vi "Periodic Tasks.vi"(0 "error in":errorcluster) -> ()   [LabVIEW 2019]
doc: "All TeleOperated, Autonomous, and Test controller logic are located here. Sensor reads and actuator commands are run inside of parallel loops. Most FRC 4265 code should be placed here."
uses:
  sensors.vi
  autoninfo.vi
  dsinstructions.vi
  constants.vi
  outputs.vi
  dsdata.vi
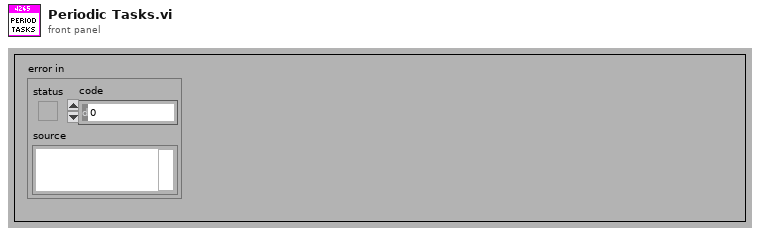
[diagram p1: front panel]
types:
  T1 = typedef "WPI_DriverStationRobotMode2.ctl" = enum16{"Autonomous Disabled", "Autonomous Enabled", "Teleop Disabled", "Teleop Enabled", "Disconnected", "Finish", "Test Disabled", "Test Enabled", "Emergency Stopped"}
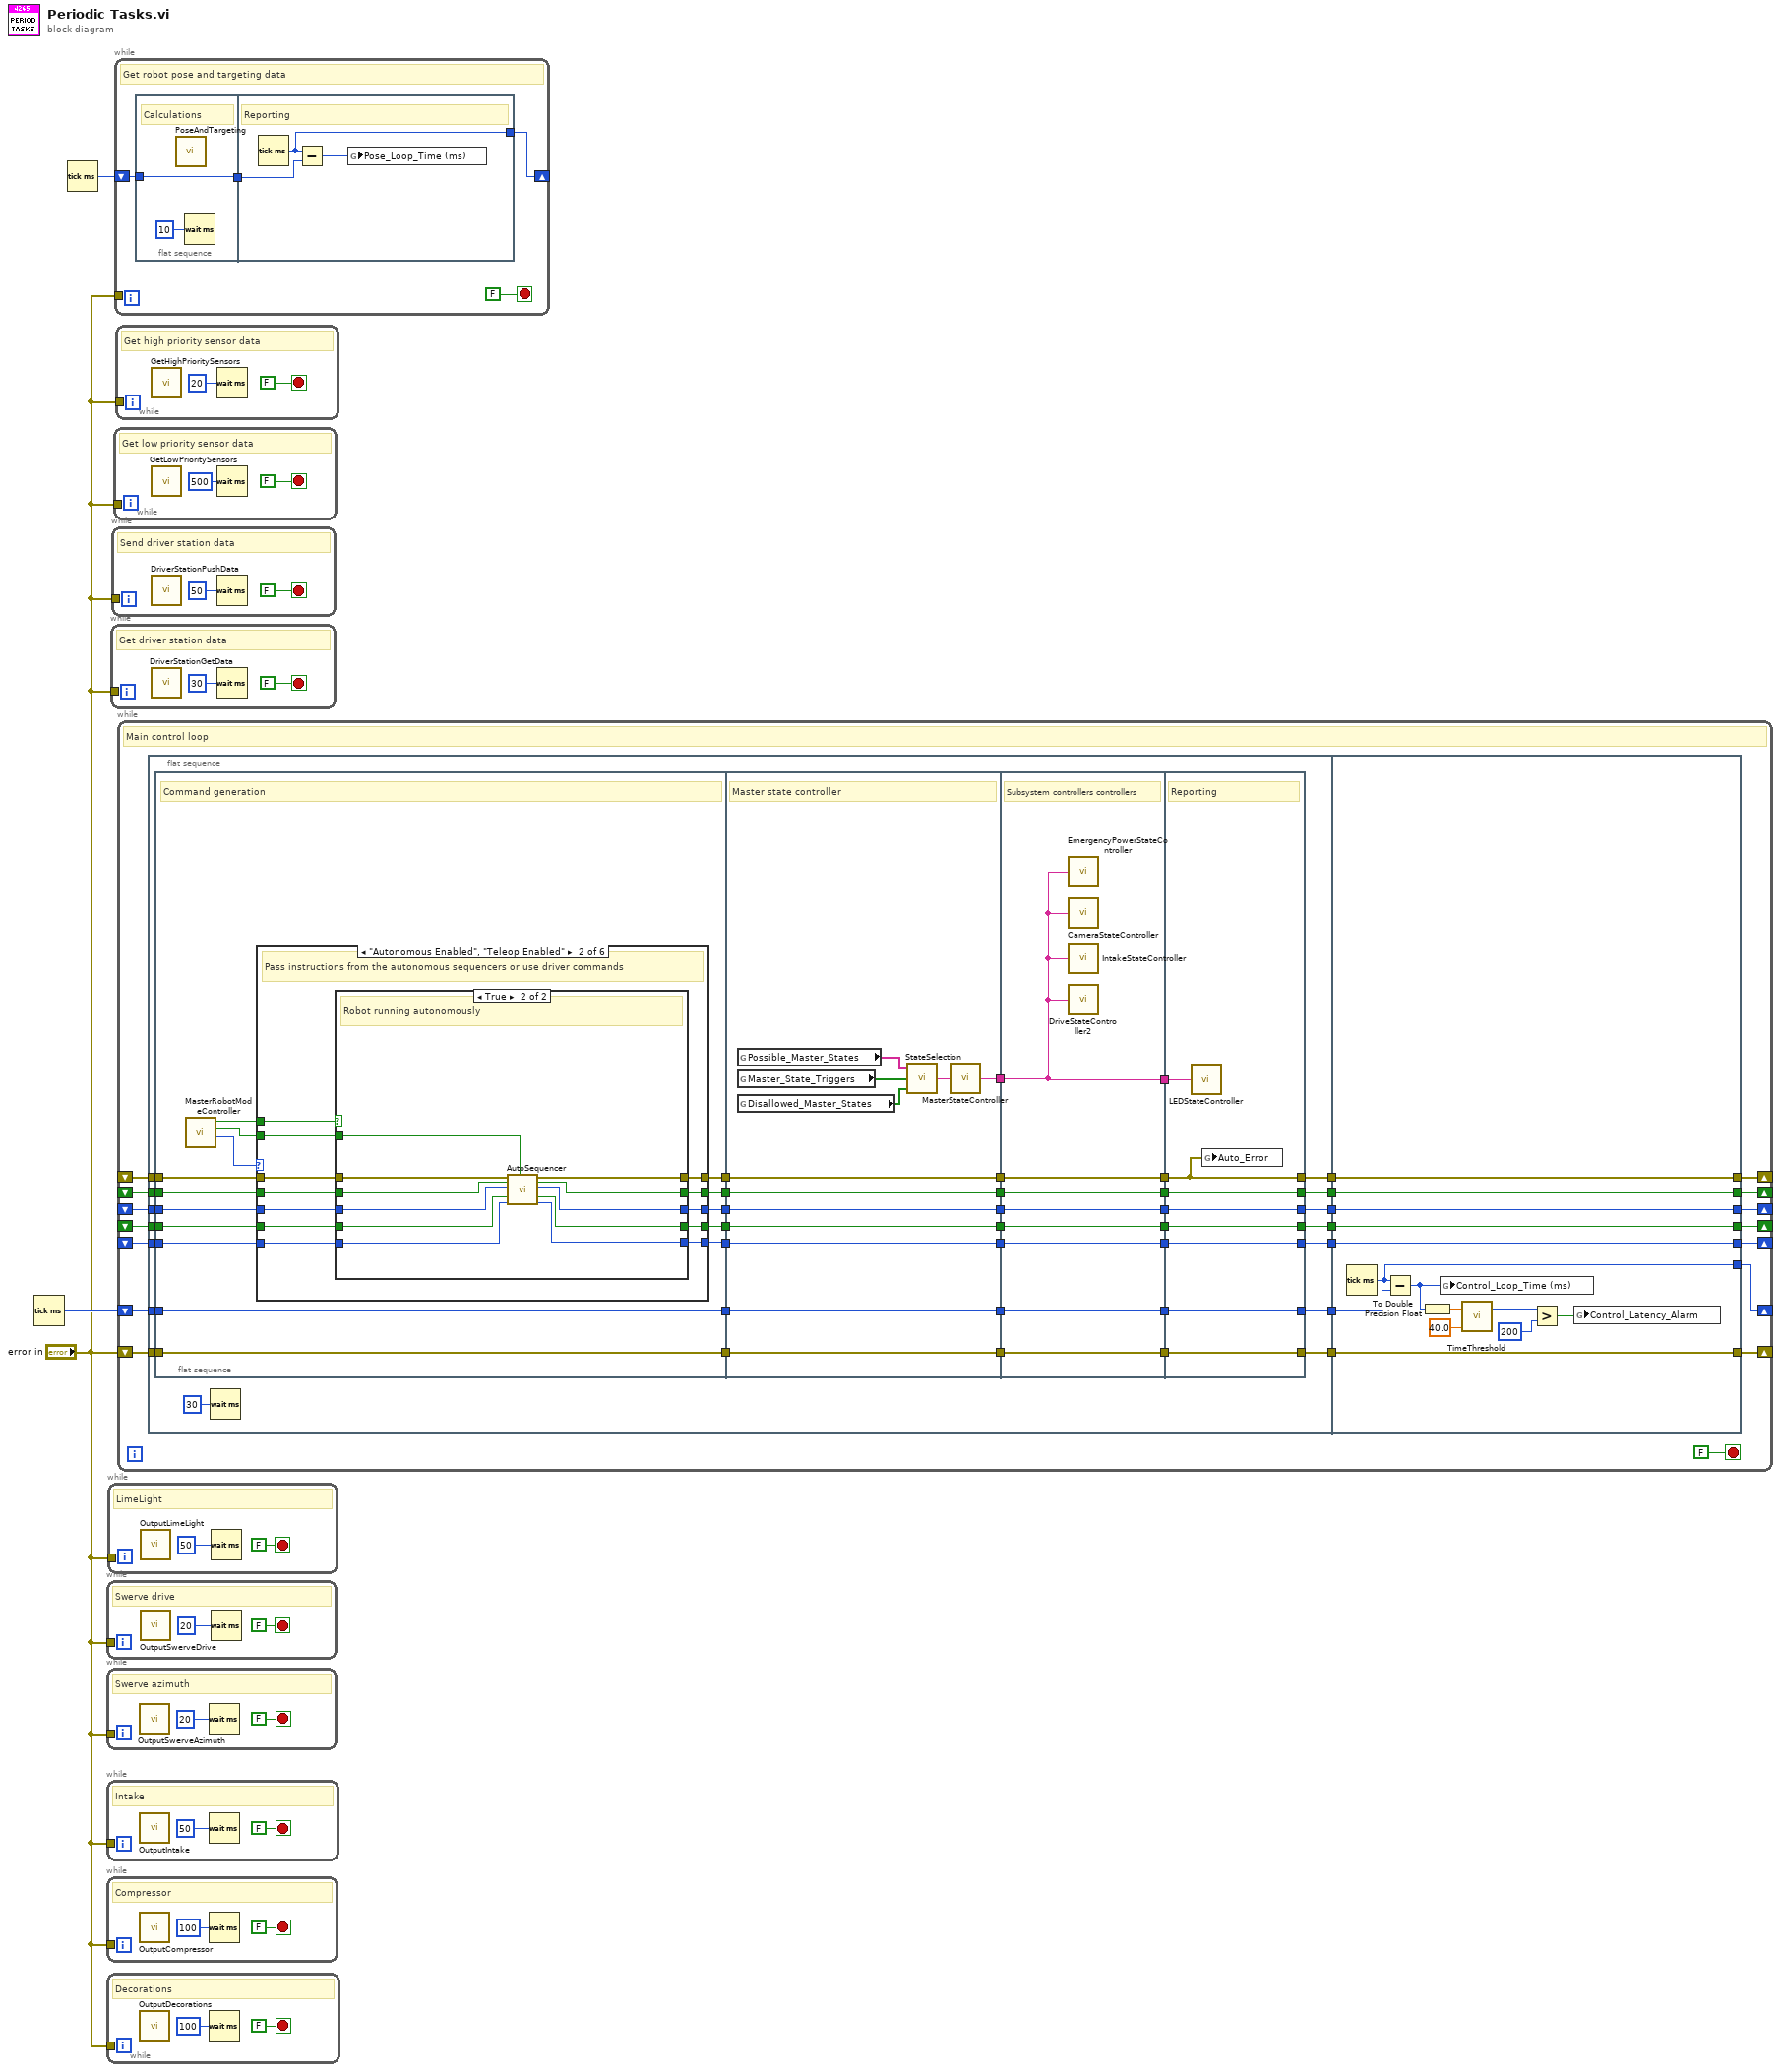
[diagram p0: block diagram]
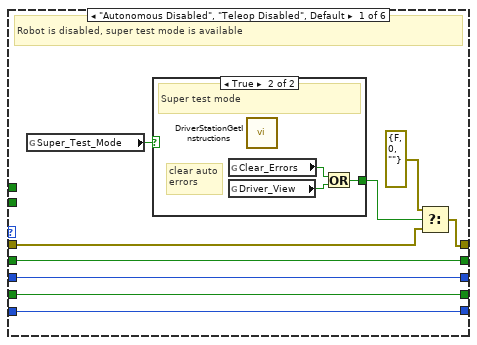
[diagram p2: hidden frame]
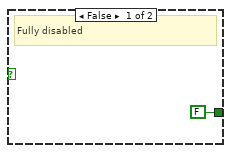
[diagram p3: hidden frame]
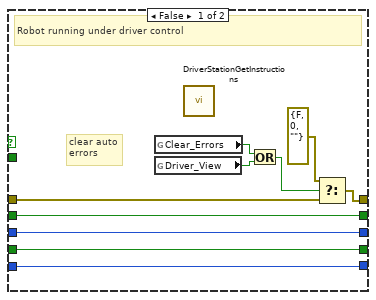
[diagram p4: hidden frame]
diagram:
  n1 = Tick Count (ms)() -> (millisecond timer value=w3:u32)
  n2 = Tick Count (ms)() -> (millisecond timer value=w1:u32)
  n3 = while {
    tunnel: "error in" -> [_]
    stop <- FALSE stop-if-true
    # "Swerve drive"
    n4 = call "OutputSwerveDrive.vi"() -> ()  [unwired: 1 in]
    n5 = Wait (ms)(milliseconds to wait=u32 20) -> ()  [unwired: 1 out]
  }
  n6 = while {
    tunnel: "error in" -> [_]
    stop <- FALSE stop-if-true
    # "Swerve azimuth"
    n7 = call "OutputSwerveAzimuth.vi"() -> ()  [unwired: 1 in]
    n8 = Wait (ms)(milliseconds to wait=u32 20) -> ()  [unwired: 1 out]
  }
  n9 = while {
    tunnel: "error in" -> [_]
    stop <- FALSE stop-if-true
    # "Intake"
    n10 = call "OutputIntake.vi"() -> ()  [unwired: 1 in]
    n11 = Wait (ms)(milliseconds to wait=u32 50) -> ()  [unwired: 1 out]
  }
  n12 = while {
    tunnel: "error in" -> [_]
    stop <- FALSE stop-if-true
    # "Compressor"
    n13 = call "OutputCompressor.vi"() -> ()  [unwired: 1 in]
    n14 = Wait (ms)(milliseconds to wait=u32 100) -> ()  [unwired: 1 out]
  }
  n15 = while {
    tunnel: "error in" -> [_]
    stop <- FALSE stop-if-true
    # "Decorations"
    n16 = call "OutputDecorations.vi"() -> ()  [unwired: 1 in]
    n17 = Wait (ms)(milliseconds to wait=u32 100) -> ()  [unwired: 1 out]
  }
  n18 = while {
    tunnel: "error in" -> [_]
    stop <- FALSE stop-if-true
    # "LimeLight"
    n19 = call "OutputLimeLight.vi"() -> ()  [unwired: 1 in]
    n20 = Wait (ms)(milliseconds to wait=u32 50) -> ()  [unwired: 1 out]
  }
  n21 = while {
    tunnel: "error in" -> [_]
    stop <- FALSE stop-if-true
    # "Get driver station data"
    n22 = call "DriverStationGetData.vi"() -> ()  [unwired: 1 in]
    n23 = Wait (ms)(milliseconds to wait=u32 30) -> ()  [unwired: 1 out]
  }
  n24 = while {
    tunnel: "error in" -> [_]
    stop <- FALSE stop-if-true
    # "Send driver station data"
    n25 = call "DriverStationPushData.vi"() -> ()  [unwired: 12 in]
    n26 = Wait (ms)(milliseconds to wait=u32 50) -> ()  [unwired: 1 out]
  }
  n27 = while {
    tunnel: "error in" -> [_]
    stop <- FALSE stop-if-true
    # "Get low priority sensor data"
    n28 = call "GetLowPrioritySensors.vi"() -> ()  [unwired: 12 in]
    n29 = Wait (ms)(milliseconds to wait=u32 500) -> ()  [unwired: 1 out]
  }
  n30 = while {
    tunnel: "error in" -> [_]
    shift-right: [w24] -> _
    shift-left: w1 -> [w23]
    stop <- FALSE stop-if-true
    # "Get robot pose and targeting data"
    n31 = flat-sequence {
      tunnel: w23 -> [w27]
      tunnel: [w27] -> w22
      tunnel: [w29] -> w24
      tunnel: w22 -> [w28]
      frame #0 {
        # "Calculations"
        n32 = call "PoseAndTargeting.vi"() -> ()  [unwired: 1 in]
        n33 = Wait (ms)(milliseconds to wait=u32 10) -> ()  [unwired: 1 out]
      }
      frame #1 {
        # "Reporting"
        n34 = Tick Count (ms)() -> (millisecond timer value=w29:u32)
        n35 = Subtract(x=w29, y=w28) -> (x-y=w30:u32)
        n36 = global write "sensors.vi" "Pose_Loop_Time (ms)"(w30) -> ()
      }
    }
  }
  n37 = while {
    tunnel: "error in" -> [_]
    stop <- FALSE stop-if-true
    # "Get high priority sensor data"
    n38 = call "GetHighPrioritySensors.vi"() -> ()  [unwired: 1 in]
    n39 = Wait (ms)(milliseconds to wait=u32 20) -> ()  [unwired: 1 out]
  }
  n40 = while {
    shift-right: [w50] -> _
    shift-left: _ -> [w52]
    shift-right: [w51] -> _
    shift-left: _ -> [w53]
    shift-right: [w49] -> _
    shift-left: _ -> [w48]
    shift-right: [w47] -> _
    shift-left: _ -> [w46]
    shift-right: [w40] -> _
    shift-left: w3 -> [w41]
    shift-right: [w45] -> _
    shift-left: _ -> [w44]
    shift-right: [w42] -> _
    shift-left: "error in" -> [w43]
    stop <- FALSE stop-if-true
    # "Main control loop"
    n41 = flat-sequence {
      tunnel: w53 -> [w69]
      tunnel: w52 -> [w68]
      tunnel: w48 -> [w64]
      tunnel: w46 -> [w62]
      tunnel: w44 -> [w60]
      tunnel: w43 -> [w59]
      tunnel: w41 -> [w57]
      tunnel: [w67] -> w39
      tunnel: [w66] -> w38
      tunnel: [w65] -> w37
      tunnel: [w63] -> w36
      tunnel: [w61] -> w35
      tunnel: [w58] -> w34
      tunnel: [w55] -> w33
      tunnel: [w202] -> w40
      tunnel: [w210] -> w42
      tunnel: [w211] -> w45
      tunnel: [w212] -> w47
      tunnel: [w213] -> w49
      tunnel: [w214] -> w50
      tunnel: [w215] -> w51
      tunnel: w39 -> [w215]
      tunnel: w38 -> [w214]
      tunnel: w37 -> [w213]
      tunnel: w36 -> [w212]
      tunnel: w35 -> [w211]
      tunnel: w34 -> [w210]
      tunnel: w33 -> [w203]
      frame #0 {
        n42 = flat-sequence {
          tunnel: w69 -> [w105]
          tunnel: w68 -> [w104]
          tunnel: [w107] -> w92
          tunnel: [w106] -> w91
          tunnel: [w103] -> w90
          tunnel: w64 -> [w102]
          tunnel: [w101] -> w89
          tunnel: w62 -> [w100]
          tunnel: [w99] -> w88
          tunnel: w60 -> [w98]
          tunnel: [w94] -> w87
          tunnel: w59 -> [w94]
          tunnel: [w93] -> w86
          tunnel: w57 -> [w93]
          tunnel: w92 -> [w174]
          tunnel: w91 -> [w185]
          tunnel: w90 -> [w184]
          tunnel: w89 -> [w183]
          tunnel: [w174] -> w85
          tunnel: [w185] -> w84
          tunnel: [w184] -> w83
          tunnel: [w183] -> w82
          tunnel: [w179] -> w81
          tunnel: [w178] -> w80
          tunnel: w88 -> [w178]
          tunnel: w87 -> [w177]
          tunnel: [w177] -> w79
          tunnel: w86 -> [w175]
          tunnel: [w175] -> w78
          tunnel: w85 -> [w193]
          tunnel: w84 -> [w192]
          tunnel: w83 -> [w191]
          tunnel: w82 -> [w190]
          tunnel: w81 -> [w186]
          tunnel: [w193] -> w77
          tunnel: [w192] -> w76
          tunnel: [w191] -> w75
          tunnel: [w190] -> w74
          tunnel: [w186] -> w73
          tunnel: [w189] -> w72
          tunnel: w80 -> [w189]
          tunnel: [w188] -> w71
          tunnel: w79 -> [w188]
          tunnel: [w187] -> w70
          tunnel: w78 -> [w187]
          tunnel: [w198] -> w63
          tunnel: [w199] -> w65
          tunnel: [w200] -> w66
          tunnel: [w201] -> w67
          tunnel: w77 -> [w201]
          tunnel: w76 -> [w200]
          tunnel: w75 -> [w199]
          tunnel: w74 -> [w198]
          tunnel: w73 -> [w197]
          tunnel: [w196] -> w61
          tunnel: w72 -> [w196]
          tunnel: [w195] -> w58
          tunnel: w71 -> [w195]
          tunnel: w70 -> [w194]
          tunnel: [w194] -> w55
          frame #0 {
            # "Command generation"
            n43 = call "MasterRobotModeController.vi"() -> ("FMS Robot Mode"=w97:T1, "Auto Reset"=w96:bool, "Robot is Autonomous"=w95:bool)  [unwired: 5 in]
            n44 = case shown="\"Autonomous Enabled\", \"Teleop Enabled\"" w97 {
              tunnel: w105 -> [w116 w129 w156 w161 w166 w171]
              tunnel: w104 -> [w115 w130 w155 w160 w165 w170]
              tunnel: [w116 w131 w156 w161 w166 w171] -> w107
              tunnel: [w115 w132 w155 w160 w165 w170] -> w106
              tunnel: w96 -> [_ w122 _ _ _ _]
              tunnel: [w114 w126 w157 w162 w167 w172] -> w103
              tunnel: w102 -> [w114 w124 w157 w162 w167 w172]
              tunnel: [w113 w125 w158 w163 w168 w173] -> w101
              tunnel: w100 -> [w113 w123 w158 w163 w168 w173]
              tunnel: [w110 w128 w154 w159 w164 w169] -> w99
              tunnel: w98 -> [w111 w127 w154 w159 w164 w169]
              tunnel: w95 -> [_ w121 _ _ _ _]
              frame "Autonomous Disabled", "Teleop Disabled", Default {
                # "Robot is disabled, super test mode is available"
                n45 = global read "dsdata.vi" "Super_Test_Mode"() -> (w112:bool)
                n46 = case shown="True" w112 {
                  tunnel: [FALSE w118] -> w108
                  frame False {
                    # "Fully disabled"
                  }
                  frame True {
                    # "clear auto\nerrors"
                    # "Super test mode"
                    n47 = global read "dsdata.vi" "Clear_Errors"() -> (w119:bool)
                    n48 = global read "dsinstructions.vi" "Driver_View"() -> (w120:bool)
                    n49 = call "DriverStationGetInstructions.vi"() -> ()  [unwired: 12 in]
                    n50 = Or(x=w119, y=w120) -> (x .or. y?=w118:bool)
                  }
                }
                n51 = Select(t=errorcluster {"status"=FALSE, "code"=0, "source"=""} ("Auto Error Out"), s=w108, f=w111) -> (s? t:f=w110:errorcluster)
              }
              frame "Autonomous Enabled", "Teleop Enabled" {
                # "Pass instructions from the autonomous sequencers or use driver commands"
                n52 = case shown="True" w121 {
                  tunnel: w122 -> [_ w145]
                  tunnel: [w133 w153] -> w132
                  tunnel: [w134 w152] -> w131
                  tunnel: w130 -> [w133 w151]
                  tunnel: w129 -> [w134 w150]
                  tunnel: [w137 w144] -> w128
                  tunnel: w127 -> [w138 w143]
                  tunnel: [w135 w149] -> w126
                  tunnel: [w136 w148] -> w125
                  tunnel: w124 -> [w135 w147]
                  tunnel: w123 -> [w136 w146]
                  frame False {
                    # "clear auto\nerrors"
                    # "Robot running under driver control"
                    n53 = global read "dsdata.vi" "Clear_Errors"() -> (w140:bool)
                    n54 = global read "dsinstructions.vi" "Driver_View"() -> (w141:bool)
                    n55 = call "DriverStationGetInstructions.vi"() -> ()  [unwired: 12 in]
                    n56 = Or(x=w140, y=w141) -> (x .or. y?=w142:bool)
                    n57 = Select(t=errorcluster {"status"=FALSE, "code"=0, "source"=""} ("Auto Error Out"), s=w142, f=w138) -> (s? t:f=w137:errorcluster)
                  }
                  frame True {
                    # "Robot running autonomously"
                    n58 = call "AutoSequencer.vi"("Auto Error In"=w143, "Mobility Advance In"=w146, "Mobility Step In"=w147, "Subsystem Advance In"=w150, "Subsystem Step In"=w151, "Reinit Sequencer"=w145) -> ("Auto Error Out"=w144:errorcluster, "Mobility Advance Out"=w148:bool, "Mobility Step Out"=w149:i32, "Subsystem Advance Out"=w152:bool, "Subsystem Step Out"=w153:i32)  [unwired: 9 in]
                  }
                }
              }
              frame "Finish" {
                # "Clean up operations are in the Finish.vi in RobotMain.vi"
              }
              frame "Test Disabled", "Test Enabled" {
                # "Use TestActuatorInterlock.vi for implimenting test code"
              }
              frame "Disconnected" {
                # "Communications have failed"
              }
              frame "Emergency Stopped" {
                # "Robot has been emergency stopped"
              }
            }
          }
          frame #1 {
            # "Master state controller"
            n59 = global read "constants.vi" "Possible_Master_States"() -> (w181:string[])
            n60 = global read "dsinstructions.vi" "Master_State_Triggers"() -> (w182:bool[])
            n61 = global read "outputs.vi" "Disallowed_Master_States"() -> (w176:bool[])
            n62 = call "StateSelection.vi"("Disallowed States"=w176, "State Triggers"=w182, "State Names"=w181) -> ("Selected State"=w180:string)
            n63 = call "MasterStateController.vi"("Selected State (In)"=w180) -> ("Selected State (Out)"=w179:string)
          }
          frame #2 {
            # "Subsystem controllers controllers"
            n64 = call "EmergencyPowerStateController.vi"("Selected State (In)"=w186) -> ()  [unwired: 1 out]
            n65 = call "CameraStateController.vi"("Selected State (In)"=w186) -> ()  [unwired: 1 out]
            n66 = call "IntakeStateController.vi"("Selected State (In)"=w186) -> ()  [unwired: 1 out]
            n67 = call "DriveStateController2.vi"("Selected State (In)"=w186) -> ()  [unwired: 1 out]
          }
          frame #3 {
            # "Reporting"
            n68 = call "LEDStateController.vi"("Selected State (In)"=w197) -> ()  [unwired: 1 out]
            n69 = global write "autoninfo.vi" "Auto_Error"(w196) -> ()
          }
        }
        n70 = Wait (ms)(milliseconds to wait=u32 30) -> ()  [unwired: 1 out]
      }
      frame #1 {
        n71 = Tick Count (ms)() -> (millisecond timer value=w202:u32)
        n72 = Subtract(x=w202, y=w203) -> (x-y=w209:u32)
        n73 = To Double Precision Float(number=w209) -> (double precision float=w208:dbl)
        n74 = global write "sensors.vi" "Control_Loop_Time (ms)"(w209) -> ()
        n75 = call "TimeThreshold.vi"("Threshold"=40.0, "Current Value"=w208) -> ("Time Above Threshold (ms)"=w207:u32)  [unwired: 1 out]
        n76 = Greater?(x=w207, y=u32 200) -> (0:w206:bool)
        n77 = global write "sensors.vi" "Control_Latency_Alarm"(w206) -> ()
      }
    }
  }
